vi "kickForceFromDistance.vi"(0 "KickToSkill in":refnum<class "KickToSkill.lvclass">, 1 "distance":dbl format="%#_13g", 2 "chipKick ?":bool, 3 "Game":refnum<class "Game.lvclass">, 4 "pass?":bool=TRUE, 5 "error in (no error)":errorcluster, 6 "shootState?":bool, 7 "KickForce":dbl, 8 "use criteria?":bool, 10 "EnableWeakKick?":bool=TRUE, 11 "Robot":refnum<class "Robot.lvclass">, 13 "multiplicativeFactorToPassForce":dbl) -> (14 "KickToSkill out":refnum<class "KickToSkill.lvclass">, 15 "kick_x Force out":dbl, 16 "kick_z Force out":dbl, 19 "error out":errorcluster)   [LabVIEW 2023, in "KickToSkill.lvclass"]
uses:
  KickToSkill.lvclass
  Game_class/Game.lvclass
  Robot_class/Robot.lvclass
  Game_class/Game.lvclass/Game.ctl
  Parameters_class/Parameters.lvclass/Parameters.ctl
  Robot_class/Robot.lvclass/Robot.ctl
  Object_class/Object.lvclass/Object.ctl
  Robot_class/Read dest_x_kick.vi
  Robot_class/Read dest_y_kick.vi
  Object_class/Read position(x,y).vi
  Game_class/Read Parameters.lvclass.vi
  Parameters_class/Read ShootOutForce.vi
  Parameters_class/Parameters.lvclass
panel:
  in  "y":dbl=3.0 format="%#_13g"
  in  "PassForceMean(default)":dbl[][](array[numeric])=[[7290.431216910258, 40.0, 0.0], [5588.112993733975, 38.0, 1.0], [3875.3759268249646, 36.0, 2.0], [2774.3232323929033, 34.0, 3.0], [1734.3636422844513, 32.0, 4.0], [1245.8077164192352, 30.0, 5.0], [999.2424946413078, 28.0, 6.0], [814.8573524752643, 26.0, 7.0], [0.0, 24.0, -1.0]]
  in  "KickForceMean(default)":dbl[][](array[numeric])=[[4656.29801400436, 70.0, 0.0], [4335.279054852332, 65.0, 1.0], [3230.618228702577, 60.0, 2.0], [2278.855764894509, 55.0, 3.0], [1340.6494904493466, 50.0, 4.0], [0.0, 45.0, -1.0]]
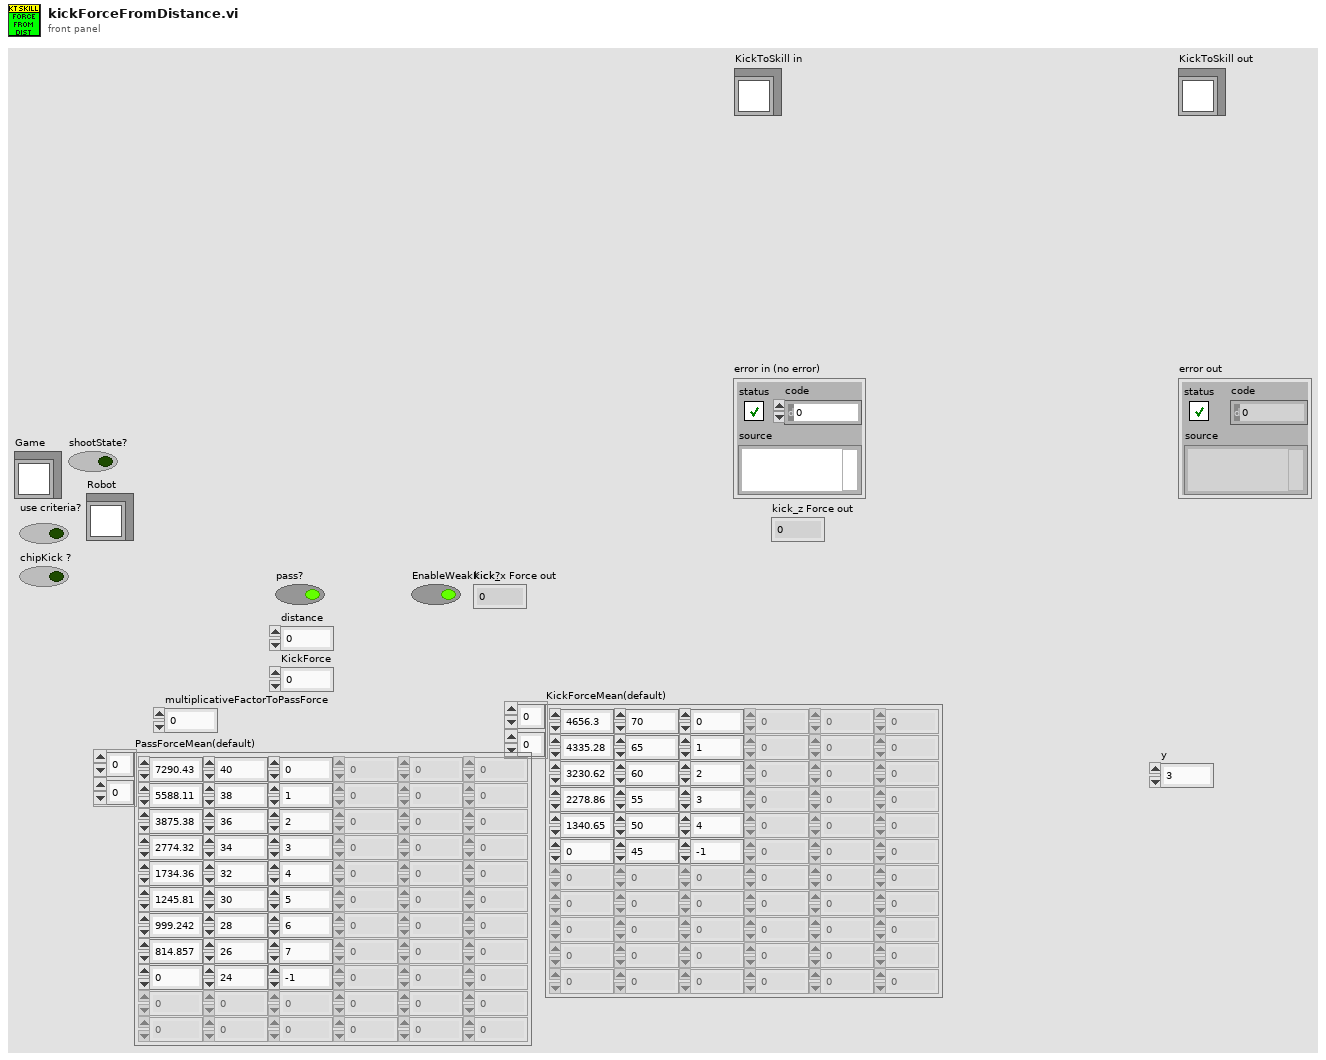
[diagram p1: front panel]
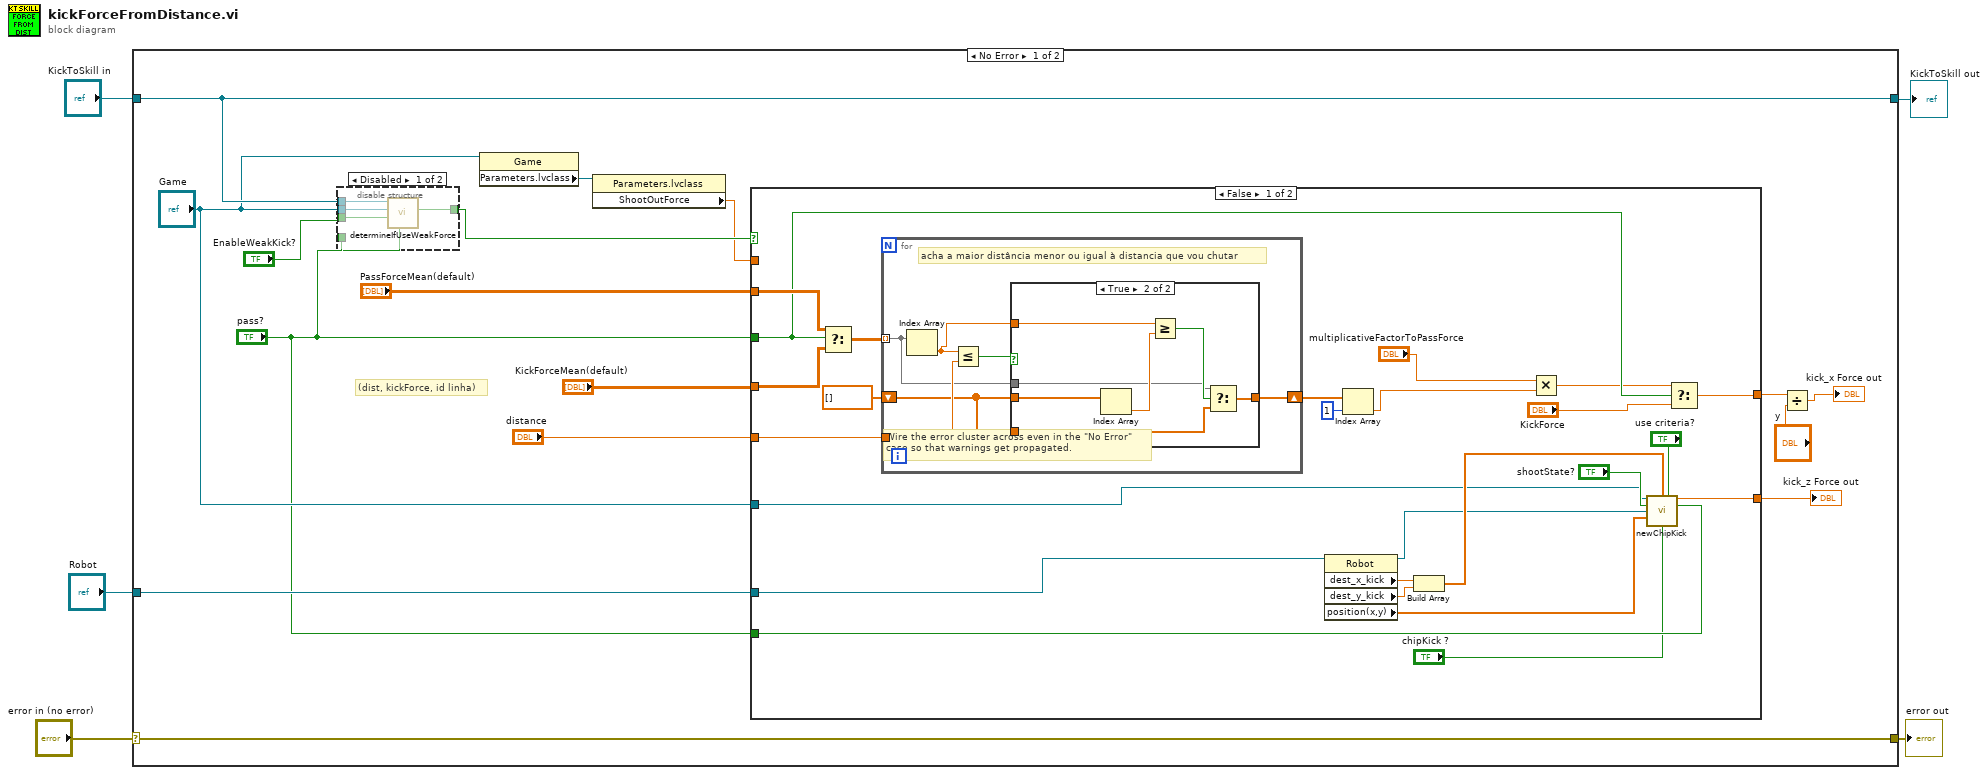
[diagram p0: block diagram]
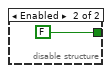
[diagram p2: hidden frame]
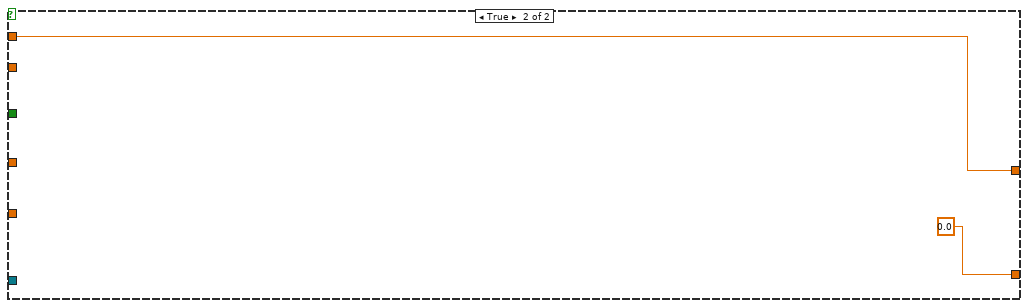
[diagram p4: hidden frame]
diagram:
  n1 = case shown="No Error" "error in (no error)" {
    selector: "error in (no error)" -> [w21 w70]
    tunnel: [w21 w70] -> w4
    tunnel: [w17 w69] -> w2
    tunnel: "KickToSkill in" -> [w17 w69]
    tunnel: "Robot" -> [w11 _]
    frame No Error {
      # "(dist, kickForce, id linha)"
      # "Wire the error cluster across even in the \"No Error\"\ncase so that warnings get propagated."
      n2 = disable-structure shown="Disabled" {
        disable-tunnel: w17 -> [w26 _]
        disable-tunnel: "EnableWeakKick?" -> [w25 _]
        disable-tunnel: [w24 FALSE ("canWeakKick")] -> w15
        disable-tunnel: "Game" -> [w23 _]
        disable-tunnel: "pass?" -> [w22 _]
        frame Disabled {
          n3 = call "determineIfUseWeakForce.vi"("pass?"=w22, "EnableWeakKick"=w25, "Game"=w23, "KickToSkill in"=w26) -> ("canWeakKick"=w24:bool)  [unwired: 5 in, 2 out]
        }
        frame Enabled {
        }
      }
      n4 = property class="Game"(reference="Game") -> ("Parameters.lvclass"=w14:refnum<class "Parameters.lvclass">)  [unwired: 1 in, 2 out]
      n5 = property class="Parameters.lvclass"(reference=w14) -> ("ShootOutForce"=w13:dbl)  [unwired: 1 in, 2 out]
      n6 = case shown="False" w15 {
        tunnel: "PassForceMean(default)" -> [w52 _]
        tunnel: "KickForceMean(default)" -> [w51 _]
        tunnel: "distance" -> [w49 _]
        tunnel: "pass?" -> [w43 _]
        tunnel: [w40 w68] -> w8
        tunnel: w13 -> [_ w68]
        tunnel: [w39 0.0] -> w9
        tunnel: "Game" -> [w29 _]
        tunnel: w11 -> [w36 _]
        tunnel: "pass?" -> [w31 _]
        frame False {
          n7 = Select(t=w52, s=w43, f=w51) -> (s? t:f=w50:dbl[][])
          n8 = for {
            tunnel: w50 -> [w55] mode=indexing
            tunnel: w49 -> [w58]
            shift-right: [w53] -> w47
            shift-left: dbl[] [] ("KickForceMean(default)") -> [w54]
            # "acha a maior distância menor ou igual à distancia que vou chutar"
            n9 = Index Array(array=w55) -> (element=w56:dbl)  [unwired: 1 in]
            n10 = Less Or Equal?(x=w56, y=w58) -> (x <= y?=w57:bool)
            n11 = case shown="True" w57 {
              tunnel: w54 -> [w59 w66]
              tunnel: w56 -> [_ w65]
              tunnel: w55 -> [_ w62]
              tunnel: w54 -> [_ w61]
              tunnel: [w59 w60] -> w53
              frame False {
              }
              frame True {
                n12 = Index Array(array=w66) -> (element=w64:dbl)  [unwired: 1 in]
                n13 = Greater Or Equal?(x=w65, y=w64) -> (x >= y?=w63:bool)
                n14 = Select(t=w62, s=w63, f=w61) -> (s? t:f=w60:dbl[])
              }
            }
          }
          n15 = property class="Robot"(reference=w36) -> (reference out=w28:refnum<class "Robot.lvclass">, "dest_x_kick"=w34:dbl, "dest_y_kick"=w33:dbl, "position(x,y)"=w35:dbl[])  [unwired: 1 in, 1 out]
          n16 = Index Array(array=w47, index=1) -> (element=w45:dbl)
          n17 = Build Array(w34, w33) -> (w32:dbl[])
          n18 = Multiply(x="multiplicativeFactorToPassForce", y=w45) -> (x*y=w42:dbl)
          n19 = call "newChipKick.vi"("Game"=w29, "Target"=w32, "use criteria?"="use criteria?", "shootState?"="shootState?", "pass ?"=w31, "Robot"=w28, "Robot Pos"=w35, "chipKick ?"="chipKick ?") -> ("ChipKick Force"=w39:dbl)  [unwired: 7 in]
          n20 = Select(t=w42, s=w43, f="KickForce") -> (s? t:f=w40:dbl)
        }
        frame True {
        }
      }
      "kick_z Force out" <- w9
      n21 = Divide(x=w8, y="y") -> (x/y=→"kick_x Force out":dbl)
    }
    frame Error {
    }
  }
  "error out" <- w4
  "KickToSkill out" <- w2
